vi "Write Update Events.vi"(8 "error in (no error)":errorcluster, 10 "Update Events":T1, 11 "CS++SimMotor in":refnum<class "CS++SimMotor.lvclass">) -> (0 "error out":errorcluster, 3 "CS++SimMotor out":refnum<class "CS++SimMotor.lvclass">)   [LabVIEW 2015, in "CS++SimMotor.lvlib" / "CS++SimMotor.lvclass"]
uses:
  CS++SimMotor.lvclass
  CS++SimMotor.lvclass/CS++SimMotor.ctl
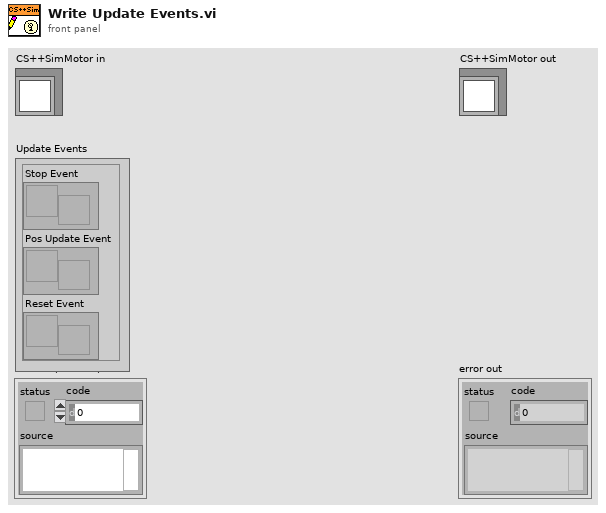
[diagram p1: front panel]
types:
  T1 = cluster{"Stop Event":refnum<user-event>, "Pos Update Event":refnum<user-event>, "Reset Event":refnum<user-event>}
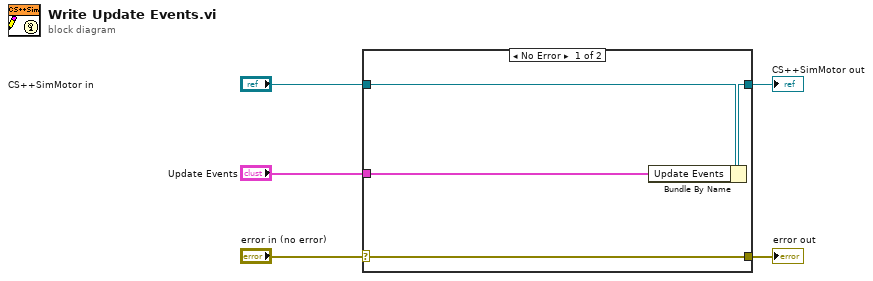
[diagram p0: block diagram]
diagram:
  n1 = case shown="No Error" "error in (no error)" {
    selector: "error in (no error)" -> [w9 w10]
    tunnel: [w9 w10] -> w4
    tunnel: [w7 w11] -> w2
    tunnel: "CS++SimMotor in" -> [w8 w11]
    tunnel: "Update Events" -> [w6 _]
    frame No Error {
      n2 = Bundle By Name(cluster=w8, "Update Events"=w6) -> (w7:refnum<class "CS++SimMotor.lvclass">)
    }
    frame Error {
    }
  }
  "error out" <- w4
  "CS++SimMotor out" <- w2
